vi "setData.vi"(8 "error in (no error)":errorcluster, 10 "data":string[][][](array[string]), 11 "reference in":refnum<class "Items Controller.lvclass">) -> (0 "error out":errorcluster, 3 "reference out":refnum<class "Items Controller.lvclass">)   [LabVIEW 2015, in "Items Controller.lvclass"]
uses:
  Items Controller.lvclass
  APP/excelFile_class/fileType.ctl
  File Controller_llb/File Controller.lvclass
  APP/excelFile_class/excelFile.lvclass
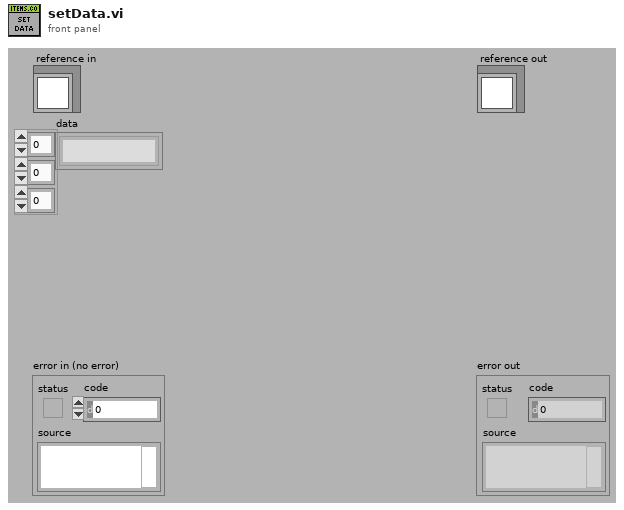
[diagram p1: front panel]
types:
  T1 = typedef "excelFile.lvclass/fileType.ctl" = enum16{"devices", "items", "partsTracking", "TSR"}
  T2 = typedef "Items Controller.lvclass/ObjectAttributesRef.ctl" = refnum<data-value>
  T3 = typedef "Items Controller.lvclass/ObjectAttributes.ctl" = cluster{"MyAttribute":dbl, "data":string[][][], "file_controller_ref":refnum<class "File Controller.lvclass">, "checkIN_ref":refnum<class "checkIN.lvclass">, "checkOUT_ref":refnum<class "checkOUT.lvclass">, "item_ref":refnum<class "item.lvclass">}
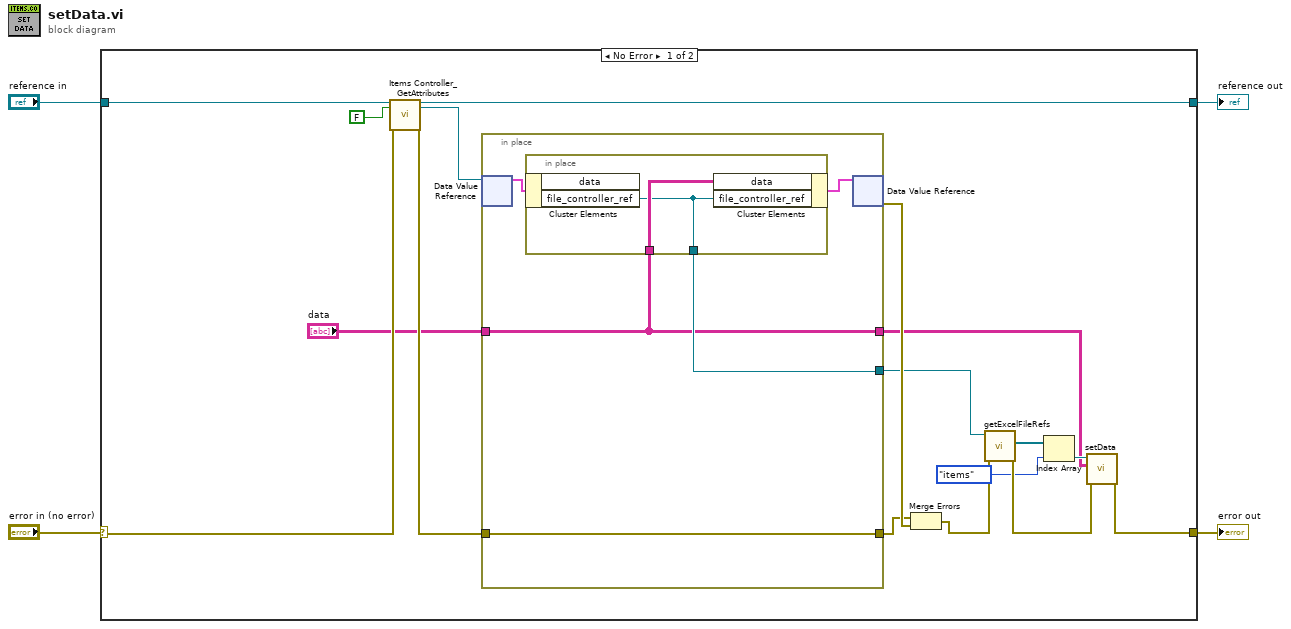
[diagram p0: block diagram]
diagram:
  n1 = case shown="No Error" "error in (no error)" {
    selector: "error in (no error)" -> [w17 w30]
    tunnel: [w9 w30] -> w3
    tunnel: [w15 w29] -> w1
    tunnel: "reference in" -> [w19 w29]
    frame No Error {
      n2 = call "Items Controller_GetAttributes.vi"("reference in"=w19, "return data? (T)"=FALSE, "error in (no error)"=w17) -> ("reference out"=w15:refnum<class "Items Controller.lvclass">, "attributes ref"=w14:T2, "error out"=w16:errorcluster)  [unwired: 13 in, 1 out]
      n3 = in-place {
        in-place-border: w16 -> [w24]
        in-place-border: [w24] -> w20
        in-place-border: "data" -> [w22]
        in-place-border: [w23] -> w12
        in-place-border: [w22] -> w6
        n4 = in-place-dvr #1(w14) -> (w25:T3)  [unwired: 1 out]
        n5 = in-place {
          in-place-border: w22 -> [w28]
          in-place-border: [w27] -> w23
          n6 = in-place-cluster #2(w25) -> ("file_controller_ref"=w27:refnum<class "File Controller.lvclass">)  [unwired: 1 out]
          n7 = in-place-cluster #2("data"=w28, "file_controller_ref"=w27) -> (w26:T3)
        }
        n8 = in-place-dvr #1(w26) -> (w21:errorcluster)  [unwired: 1 out]
      }
      n9 = Merge Errors(w20, w21) -> (w11:errorcluster)
      n10 = call "getExcelFileRefs.vi"("error in (no error)"=w11, "reference in"=w12) -> ("error out"=w10:errorcluster, "excelFile_refs"=w8:refnum<class "excelFile.lvclass">[])  [unwired: 7 in, 1 out]
      n11 = Index Array(array=w8, index=fileType."items" ("fileType")) -> (element=w7:refnum<class "excelFile.lvclass">)
      n12 = call "setData.vi"("error in (no error)"=w10, "data"=w6, "reference in"=w7) -> ("error out"=w9:errorcluster)  [unwired: 7 in, 1 out]
    }
    frame Error {
    }
  }
  "error out" <- w3
  "reference out" <- w1
